vi "实时数据发送 (子VI).vi"(11 "数值":i32) -> (3 "超时退出":bool)   [LabVIEW 2016, in "数据传输系统-06.lvlib"]
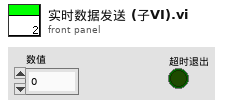
[diagram p1: front panel]
types:
  T1 = typedef "数据传输系统-06.lvlib/应用环境.ctl" = enum16{"STD", "GB212", "婉仪平台"}
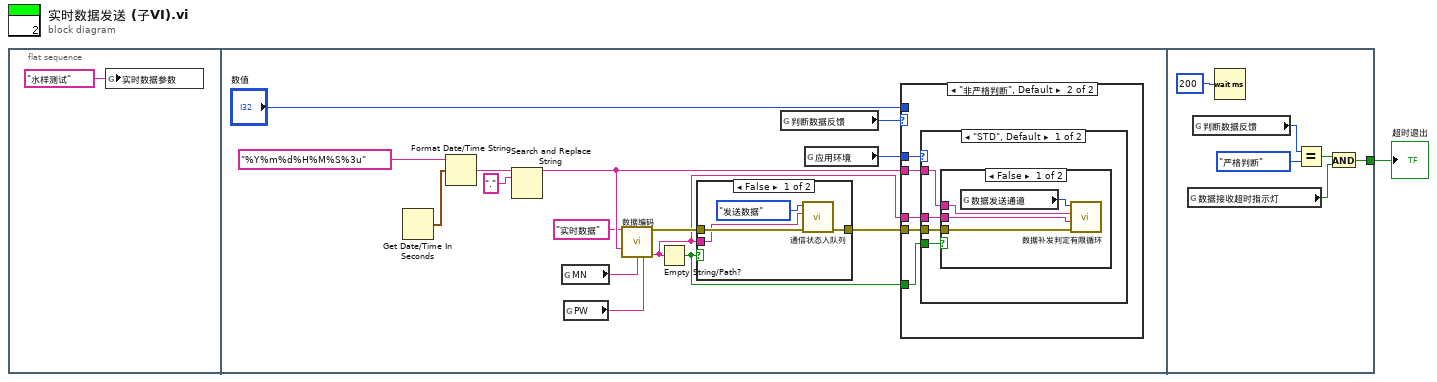
[diagram p0: block diagram]
diagram:
  n1 = flat-sequence {
    tunnel: [w36] -> w1
    frame #0 {
      n2 = global write "全局 实时数据参数.vi" "实时数据参数"("水样测试" ("实时数据参数")) -> ()
    }
    frame #1 {
      n3 = Get Date/Time In Seconds() -> (seconds since 1Jan1904=w15:timestamp)
      n4 = Format Date/Time String(time format string (%c)="%Y%m%d%H%M%S%3u" ("时间格式字符串(%c)"), seconds (now)=w15) -> (date/time string=w14:string)  [unwired: 1 in]
      n5 = Search and Replace String(input string=w14, search string="." ("搜索字符串")) -> (result string=w17:string)  [unwired: 6 in, 3 out]
      n6 = global read "断电保存全局.vi" "MN"() -> (w9:string)
      n7 = global read "断电保存全局.vi" "PW"() -> (w10:string)
      n8 = call "数据编码.vi"("table输入"="实时数据" ("新元素/子数组"), "QN"=w17, "MN"=w9, "PW"=w10) -> ("错误常量"=w8:errorcluster, "通讯包字符串"=w4:string)  [unwired: 10 in]
      n9 = Empty String/Path?(string/path=w4) -> (empty?=w3:bool)
      n10 = case shown="False" w3 {
        tunnel: [w21 w22] -> w11
        tunnel: w8 -> [w20 w22]
        tunnel: w4 -> [w18 _]
        frame False {
          n11 = call "通信状态入队列.vi"("错误输入（无错误）"=w20, "发送报文"=w18, "枚举"=enum16{"打开连接", "发送数据", "读取数据", "数据处理", "关闭连接"}."发送数据") -> ("错误输出"=w21:errorcluster)  [unwired: 8 in]
        }
        frame True {
        }
      }
      n12 = global read "断电保存全局.vi" "判断数据反馈"() -> (w12:enum16{"非严格判断", "严格判断", "不判断"})
      n13 = global read "断电保存全局.vi" "应用环境"() -> (w5:T1)
      n14 = case shown="\"非严格判断\", Default" w12 {
        tunnel: w4 -> [_ w27]
        tunnel: w11 -> [_ w26]
        tunnel: "数值" -> [_ _]
        tunnel: w17 -> [_ w25]
        tunnel: w5 -> [_ w24]
        tunnel: w3 -> [_ w23]
        frame "不判断" {
        }
        frame "非严格判断", Default {
          n15 = case shown="\"STD\", Default" w24 {
            tunnel: w27 -> [w29 _]
            tunnel: w26 -> [w31 _]
            tunnel: w25 -> [w30 _]
            tunnel: w23 -> [w28 _]
            frame "STD", Default {
              n16 = case shown="False" w28 {
                tunnel: w31 -> [w35 _]
                tunnel: w30 -> [w33 _]
                tunnel: w29 -> [w32 _]
                frame False {
                  n17 = global read "断电保存全局.vi" "数据发送通道"() -> (w34:enum16{"TCP", "VISA"})
                  n18 = call "数据补发判定有限循环.vi"("错误输入（无错误）"=w35, "数据输入"=w32, "QN"=w33, "数据发送通道"=w34) -> ()  [unwired: 7 in, 1 out]
                }
                frame True {
                }
              }
            }
            frame "GB212" {
            }
          }
        }
      }
    }
    frame #2 {
      n19 = global read "全局 数据发送重叠.vi" "数据接收超时指示灯"() -> (w37:bool)
      n20 = global read "断电保存全局.vi" "判断数据反馈"() -> (w40:enum16{"非严格判断", "严格判断", "不判断"})
      n21 = Wait (ms)(milliseconds to wait=u32 200 ("等待时间（毫秒）")) -> ()  [unwired: 1 out]
      n22 = Equal?(x=w40, y=enum16{"非严格判断", "严格判断", "不判断"}."严格判断") -> (x = y?=w38:bool)
      n23 = And(x=w38, y=w37) -> (x .and. y?=w36:bool)
    }
  }
  "超时退出" <- w1
